vi "polling_events.vi"() -> ()   [LabVIEW 2014]
uses:
  lvnanomsg/socket_options.ctl
  lvnanomsg/nanomsg_context.lvclass
  lvnanomsg/nanomsg_socket.lvclass
  lvnanomsg/nanomsg.lvlib
panel:
  out "String":string
  out "Numeric":i32
  out "error out":errorcluster
  out "messages":string[](array[string])
  in  "endpoint":string="tcp://127.0.0.1:5555"
  # "Nanomsg polling-based receive events"
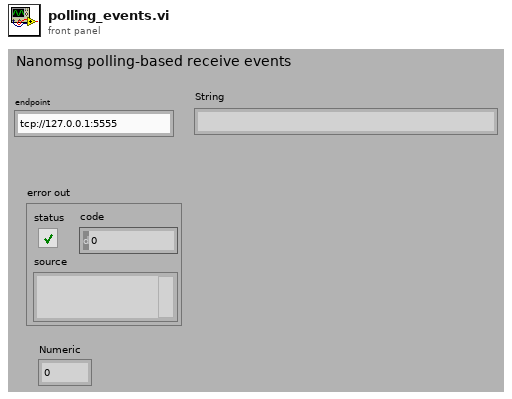
[diagram p1: front panel]
types:
  T1 = typedef "nanomsg.lvlib/socket_options.ctl" = u16
  T2 = enum16{"NN_SUB_XXX", "NN_SUB_SUBSCRIBE", "NN_SUB_UNSUBSCRIBE"}
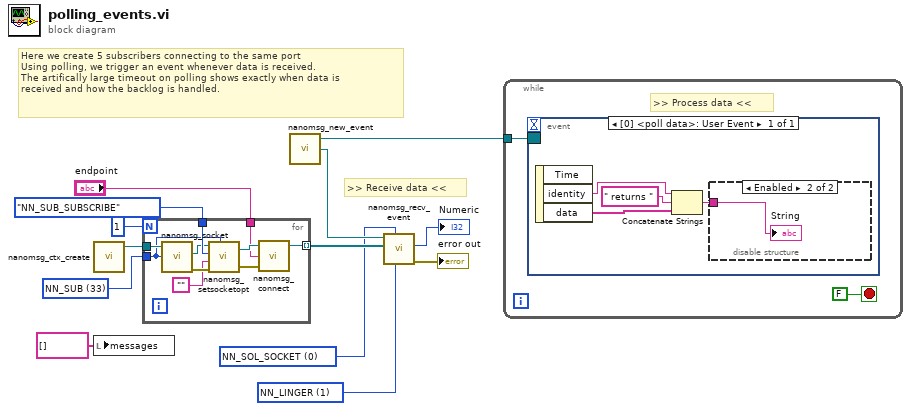
[diagram p0: block diagram]
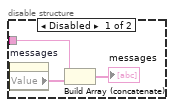
[diagram p2: hidden frame]
diagram:
  w3 = T1 1 items=["NN_LINGER"=1, "NN_SNDBUF"=2, "NN_RCVBUF"=3, "NN_SNDTIMEO"=4, "NN_RCVTIMEO"=5, "NN_RECONNECT_IVL"=6, "NN_RECONNECT_IVL_MAX"=7, "NN_SNDPRIO"=8, "NN_RCVPRIO"=9, "NN_SNDFD"=10, "NN_RCVFD"=11, "NN_DOMAIN"=12, "NN_PROTOCOL"=13, "NN_IPV4ONLY"=14, "NN_SOCKET_NAME"=15, "NN_RCVMAXSIZE"=16, "NN_MAXTTL"=17] ("Socket option")
  w4 = 0 items=["NN_WS"=-4, "NN_TCP"=-3, "NN_IPC"=-2, "NN_INPROC"=-1, "NN_SOL_SOCKET"=0, "NN_PAIR"=16, "NN_PUB"=32, "NN_SUB"=33, "NN_REQ"=48, "NN_REP"=49, "NN_PUSH"=80, "NN_PULL"=81, "NN_SURVEYOR"=98, "NN_RESPONDENT"=99, "NN_BUS"=112] ("socket type")
  w6 = 33 items=["NN_WS"=-4, "NN_TCP"=-3, "NN_IPC"=-2, "NN_INPROC"=-1, "NN_SOL_SOCKET"=0, "NN_PAIR"=16, "NN_PUB"=32, "NN_SUB"=33, "NN_REQ"=48, "NN_REP"=49, "NN_PUSH"=80, "NN_PULL"=81, "NN_SURVEYOR"=98, "NN_RESPONDENT"=99, "NN_BUS"=112] ("socket type")
  # "Here we create 5 subscribers connecting to the same port\nUsing polling, we trigger an event whenever data is received.\nThe artifically large timeout on polling shows exactly when data is\nreceived and how the backlog is handled."
  # ">> Receive data <<"
  n1 = call "nanomsg_ctx_create.vi"() -> ("context out"=w13:refnum<class "nanomsg_context.lvclass">)  [unwired: 4 in, 1 out]
  n2 = local write "messages"(string[] [] ("messages")) -> ()
  n3 = for {
    N: 1 -> [_]
    tunnel: w13 -> [w23]
    tunnel: [w22] -> w9 mode=indexing
    tunnel: T2."NN_SUB_SUBSCRIBE" ("option") -> [w20]
    tunnel: w6 -> [w14]
    tunnel: "endpoint" -> [w16]
    n4 = call "nanomsg_socket.vi"("socket type"=w14, "context in"=w23) -> ("error out"=w21:errorcluster, "socket out"=w15:refnum<class "nanomsg_socket.lvclass">)  [unwired: 3 in, 1 out]
    n5 = call "nanomsg_setsocketopt.vi"("socket in"=w15, "option"=w20, "value"="", "error in"=w21, "level"=w14) -> ("socket out"=w18:refnum<class "nanomsg_socket.lvclass">, "error out"=w17:errorcluster)
    n6 = call "nanomsg_connect.vi"("error in"=w17, "endpoint"=w16, "socket in"=w18) -> ("socket out"=w22:refnum<class "nanomsg_socket.lvclass">)  [unwired: 1 in, 1 out]
  }
  n7 = call "nanomsg_new_event.vi"() -> ("user event"=w7:refnum<user-event>, "event ref out"=w8:refnum<event-registration>)  [unwired: 3 in, 1 out]
  n8 = call "nanomsg_recv_event.vi"("options"=w3, "level"=w4, "sockets"=w9, "poll event"=w7) -> ("error out"=→"error out":errorcluster, "nevents"=→"Numeric":i32)  [unwired: 3 in, 1 out]
  n9 = while {
    tunnel: w8 -> [w25]
    stop <- FALSE stop-if-true
    # ">> Process data <<"
    n10 = event shown="[0] <poll data>: User Event" {
      selector: w25 -> [_]
      dyn-events: _ -> [_]
      timeout: _ -> [_]
      event User Event {
        n11 = event-data() -> ("identity"=w26:string, "data"=w27:string[])  [unwired: 1 in, 1 out]
        n12 = Concatenate Strings(w26, " returns " ("string"), w27) -> (w29:string)
        n13 = disable-structure shown="Enabled" {
          disable-tunnel: w29 -> [w31 w33]
          frame Disabled {
            n14 = property on="messages" class="Arr (strict)"() -> ("Value"=w30:string[])  [unwired: 2 in, 2 out]
            n15 = Build Array (concatenate)(w31, w30) -> (→"messages":string[])
          }
          frame Enabled {
            "String" <- w33
          }
        }
      }
    }
  }
